vi "FL_Make_data_frame_and_put_to_queue_2.vi"(8 "error in":errorcluster, 10 "Queue in":refnum<queue>, 11 "VISA resource name in":refnum<visa-resource-name>) -> (0 "error out":errorcluster, 2 "Queue out":refnum<queue>, 3 "VISA resource name out":refnum<visa-resource-name>, 5 "Read buffer (for reference only, data is queued)":string)   [LabVIEW 2018]
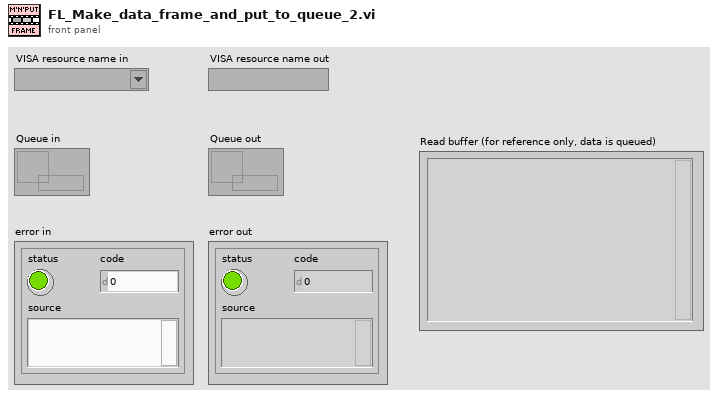
[diagram p1: front panel]
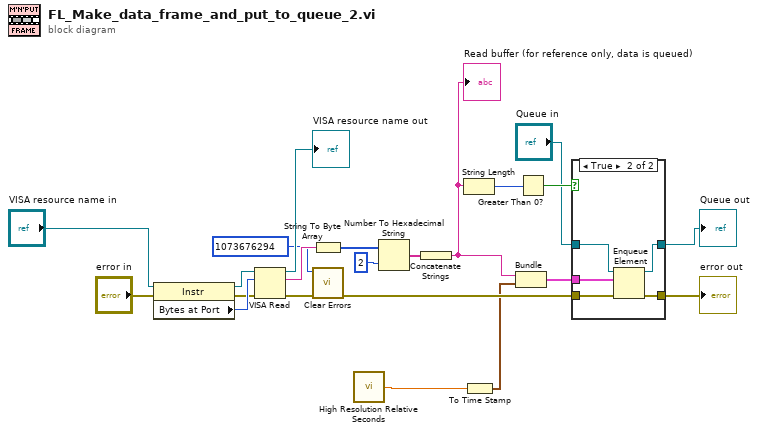
[diagram p0: block diagram]
diagram:
  n1 = property class="Instr"(reference="VISA resource name in", error in="error in") -> (reference out=w7:refnum<visa-resource-name>, error out=w8:errorcluster, "Bytes at Port"=w9:u32)
  n2 = VISA Read(VISA resource name=w7, byte count=w9, error in (no error)=w8) -> (VISA resource name out=→"VISA resource name out":refnum<visa-resource-name>, read buffer=w11:string, error out=w12:errorcluster)  [unwired: 1 out]
  n3 = String To Byte Array(string=w11) -> (unsigned byte array=w3:u8[])
  n4 = call <vilib>:"Clear Errors.vi"("error in (no error)"=w12, "specific error code to clear (0: all)"=1073676294) -> ("error out"=w20:errorcluster)  [unwired: 4 in, 1 out]
  n5 = call <vilib>:"High Resolution Relative Seconds.vi"() -> ("relative seconds"=w2:dbl)
  n6 = Number To Hexadecimal String(1:i16 2 ("width (-)"), 2:w3) -> (0:w5:string[])
  n7 = Concatenate Strings(w5) -> (w22:string)
  "Read buffer (for reference only, data is queued)" <- w22
  n8 = String Length(string=w22) -> (length=w16:i32)
  n9 = To Time Stamp(1:w2) -> (0:w1:timestamp)
  n10 = Bundle(w22, w1) -> (w19:cluster{string, timestamp})  [unwired: 1 in]
  n11 = Greater Than 0?(x=w16) -> (x > 0?=w21:bool)
  n12 = case shown="True" w21 {
    tunnel: w19 -> [_ w25]
    tunnel: w20 -> [w24 w27]
    tunnel: [w24 w26] -> w13
    tunnel: "Queue in" -> [w23 w29]
    tunnel: [w23 w28] -> w15
    frame False {
    }
    frame True {
      n13 = Enqueue Element(queue=w29, element=w25, error in (no error)=w27) -> (queue out=w28:refnum<queue>, error out=w26:errorcluster)  [unwired: 1 in, 1 out]
    }
  }
  "Queue out" <- w15
  "error out" <- w13
